vi "DigitalOutput Example.vi"() -> ()   [LabVIEW 2012, in "Phidget Digital Output.lvlib"]
uses:
  <instrlib>/Phidgets/Phidget Digital Output/Phidget Digital Output.lvlib
  <instrlib>/Phidgets/Phidget Digital Output/Public/DigitalOutputStart.vi
  <instrlib>/Phidgets/Phidget Digital Output/Public/DigitalOutputClose.vi
  <instrlib>/Phidgets/Phidget Common/Phidget Common.lvlib
panel:
  in  "LEDForwardVoltage":u32(ring) items=["LED_FORWARD_VOLTAGE_1_7V"=1, "LED_FORWARD_VOLTAGE_2_75V"=2, "LED_FORWARD_VOLTAGE_3_2V"=3, "LED_FORWARD_VOLTAGE_3_9V"=4, "LED_FORWARD_VOLTAGE_4_0V"=5, "LED_FORWARD_VOLTAGE_4_8V"=6, "LED_FORWARD_VOLTAGE_5_0V"=7, "LED_FORWARD_VOLTAGE_5_6V"=8]
  in  "Is Hub Port?":bool
  in  "error in (no error)":errorcluster
  in  "Device Info":T1={"Serial Number"=-1, "Channel"=0, "Port"=0}
  out "Attached?":bool
  in  "LED Current Limit":dbl=0.02
  in  "State":bool
  in  "DutyCycle":dbl(slide) scale=0.0..1.0
  in  "STOP":bool
  out "error out":errorcluster
  # "Yes"
  # "No"
  # "LEDForwardVoltage and LED Current Limit\nonly need to be set for dedicated LED controllers"
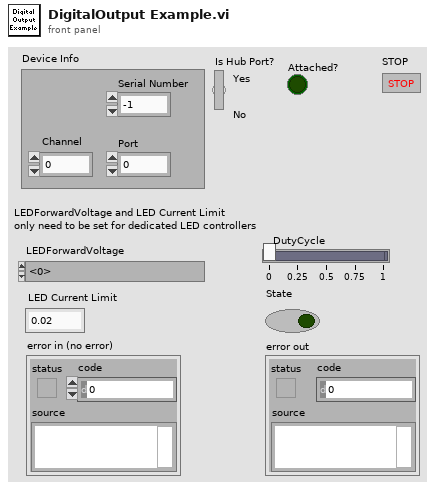
[diagram p1: front panel]
types:
  T1 = cluster{"Serial Number":i32, "Channel":i32, "Port":i32}
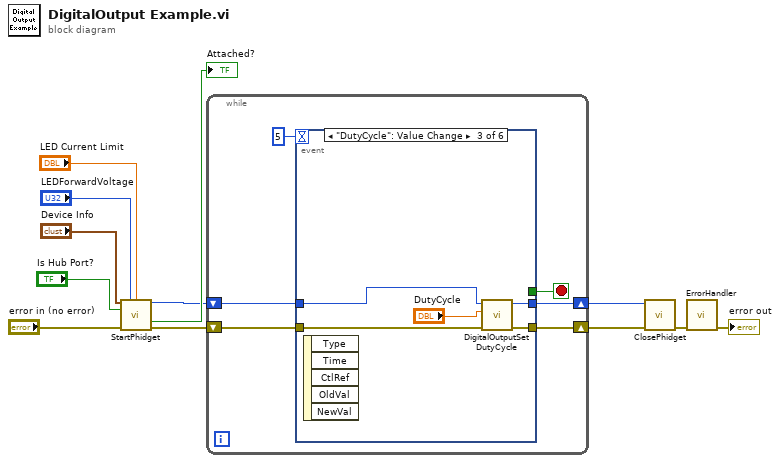
[diagram p0: block diagram]
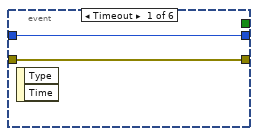
[diagram p2: hidden frame]
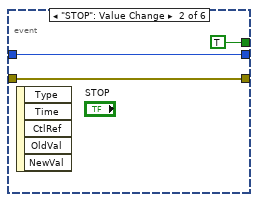
[diagram p3: hidden frame]
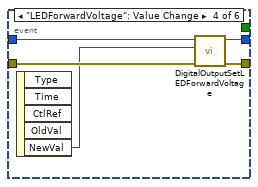
[diagram p4: hidden frame]
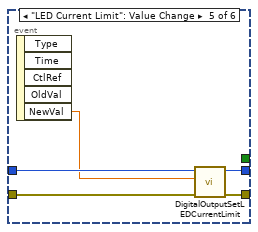
[diagram p5: hidden frame]
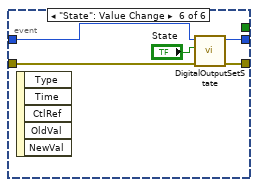
[diagram p6: hidden frame]
diagram:
  n1 = call-poly <instrlib>:"StartPhidget.vi"("Device Info"="Device Info", "LEDForwardVoltage"="LEDForwardVoltage", "Current Limit"="LED Current Limit", "IsHubPort"="Is Hub Port?", "error in (no error)"="error in (no error)") -> ("Phidget ID"=w4:u64, "Attached?"=→"Attached?":bool, "error out"=w3:errorcluster)  [unwired: 7 in, 1 out]
  n2 = while {
    shift-right: [w14] -> w9
    shift-left: w4 -> [w18]
    shift-right: [w13] -> w10
    shift-left: w3 -> [w17]
    stop <- w15 stop-if-true
    n3 = event shown="[2] \"DutyCycle\": Value Change" {
      selector: _ -> [_ _ _ _ _ _]
      dyn-events: _ -> [_ _ _ _ _ _]
      timeout: 5 -> [_ _ _ _ _ _]
      tunnel: w18 -> [w20 w22 w28 w33 w38 w43]
      tunnel: w17 -> [w19 w21 w27 w32 w37 w40]
      tunnel: [w19 w21 w25 w31 w35 w41] -> w13
      tunnel: [w20 w22 w26 w30 w36 w42] -> w14
      tunnel: [_ TRUE ("Stop") _ _ _ _] -> w15
      event Timeout {
        n4 = event-data() -> ()  [unwired: 1 in, 2 out]
      }
      event "STOP": Value Change {
        n5 = event-data() -> ()  [unwired: 1 in, 5 out]
      }
      event "DutyCycle": Value Change {
        n6 = event-data() -> ()  [unwired: 1 in, 5 out]
        n7 = call <instrlib>:"DigitalOutputSetDutyCycle.vi"("error in (no error)"=w27, "Duty Cycle"="DutyCycle", "Device In"=w28) -> ("error out"=w25:errorcluster, "Device Out"=w26:u64)  [unwired: 6 in]
      }
      event "LEDForwardVoltage": Value Change {
        n8 = event-data() -> ("NewVal"=w29:u32)  [unwired: 1 in, 4 out]
        n9 = call <instrlib>:"DigitalOutputSetLEDForwardVoltage.vi"("error in (no error)"=w32, "LEDForwardVoltage"=w29, "Device In"=w33) -> ("error out"=w31:errorcluster, "Device Out"=w30:u64)  [unwired: 6 in]
      }
      event "LED Current Limit": Value Change {
        n10 = event-data() -> ("NewVal"=w34:dbl)  [unwired: 1 in, 4 out]
        n11 = call <instrlib>:"DigitalOutputSetLEDCurrentLimit.vi"("error in (no error)"=w37, "Current Limit"=w34, "Device In"=w38) -> ("error out"=w35:errorcluster, "Device Out"=w36:u64)  [unwired: 6 in]
      }
      event "State": Value Change {
        n12 = event-data() -> ()  [unwired: 1 in, 5 out]
        n13 = call <instrlib>:"DigitalOutputSetState.vi"("error in (no error)"=w40, "State"="State", "Device In"=w43) -> ("error out"=w41:errorcluster, "Device Out"=w42:u64)  [unwired: 6 in]
      }
    }
  }
  n14 = call-poly <instrlib>:"ClosePhidget.vi"("error in"=w10, "Device In"=w9) -> ("error out"=w12:errorcluster)  [unwired: 9 in]
  n15 = call <instrlib>:"ErrorHandler.vi"("error in"=w12) -> ("error out"=→"error out":errorcluster)  [unwired: 9 in, 1 out]
